vi "MGI Determine Time Format String.vi"(8 "error in (no error)":errorcluster, 9 "Day Before Month? (F)":bool, 10 "Leading Zeros? (F)":bool, 11 "DateTime String":string) -> (0 "error out":errorcluster, 3 "DateTime Format":string)   [LabVIEW 2016]
doc: "Determines a Time Format String for a given string in a common date format. For example Thu, January 1, 2011 3:00 PM would be %a, %B, %#d, %Y %#I:%M %p. The <b>Day Before Month?</b> input specifies whether the day or month is first when in a 12/1/11 type format. The <b>Leading Zeros?</b> input determines if the day, month number, and hour will have a leading zero if they are only 1 digit.\n\nAuthored by Hope Harrison\nsupport@mooregoodideas.com\nwww.mooregoodideas.com\n\nCopyright (c) 2010, Moore Good Ideas, Inc.\n\nAll rights reserved.\n\nRedistribution and use in source and binary forms, with or without modification, are permitted provided that the following conditions are met:\n\n * Redistributions of source code must retain the above copyright notice, this list of conditions and the following disclaimer.\n * Redistributions in binary form must reproduce the above copyright notice, this list of conditions and the following disclaimer in the documentation and/or other materials provided with the distribution.\n * Neither the name of Moore Good Ideas, Inc. nor the names of its contributors may be used to endorse or promote products derived from this software without specific prior written permission.\n\nTHIS SOFTWARE IS PROVIDED BY THE COPYRIGHT HOLDERS AND CONTRIBUTORS \"AS IS\" AND ANY EXPRESS OR IMPLIED WARRANTIES, INCLUDING, BUT NOT LIMITED TO, THE IMPLIED WARRANTIES OF MERCHANTABILITY AND FITNESS FOR A PARTICULAR PURPOSE ARE DISCLAIMED. IN NO EVENT SHALL THE COPYRIGHT OWNER OR CONTRIBUTORS BE LIABLE FOR ANY DIRECT, INDIRECT, INCIDENTAL, SPECIAL, EXEMPLARY, OR CONSEQUENTIAL DAMAGES (INCLUDING, BUT NOT LIMITED TO, PROCUREMENT OF SUBSTITUTE GOODS OR SERVICES; LOSS OF USE, DATA, OR PROFITS; OR BUSINESS INTERRUPTION) HOWEVER CAUSED AND ON ANY THEORY OF LIABILITY, WHETHER IN CONTRACT, STRICT LIABILITY, OR TORT (INCLUDING NEGLIGENCE OR OTHERWISE) ARISING IN ANY WAY OUT OF THE USE OF THIS SOFTWARE, EVEN IF ADVISED OF THE POSSIBILITY OF SUCH DAMAGE."
uses:
  <userlib>/_MGI/String/MGI Determine Time Format String/MGI Local Time Strings.ctl
  <userlib>/_MGI/String/MGI Determine Time Format String/MGI Parts of Date Found.ctl
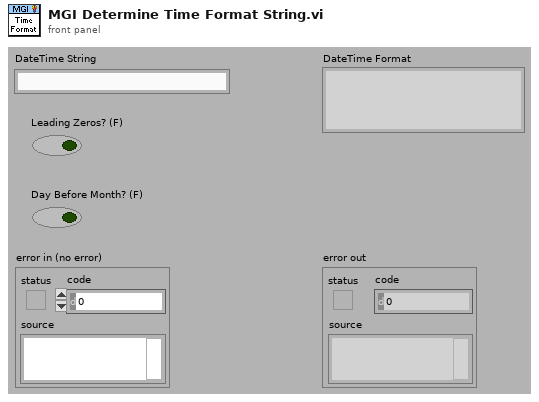
[diagram p1: front panel]
types:
  T1 = typedef "MGI Local Time Strings.ctl" = cluster{"Month[]":string[], "AMPM[]":string[], "Weekday[]":string[]}
  T2 = cluster{"fractional second":dbl, "second":i32, "minute":i32, "hour":i32, "day of month":i32, "month":i32, "year":i32, "day of week":i32, "day of year":i32, "DST":i32}
  T3 = typedef "MGI Parts of Date Found.ctl" = cluster{"Found Month?":bool, "Found Day?":bool, "Found Year?":bool}
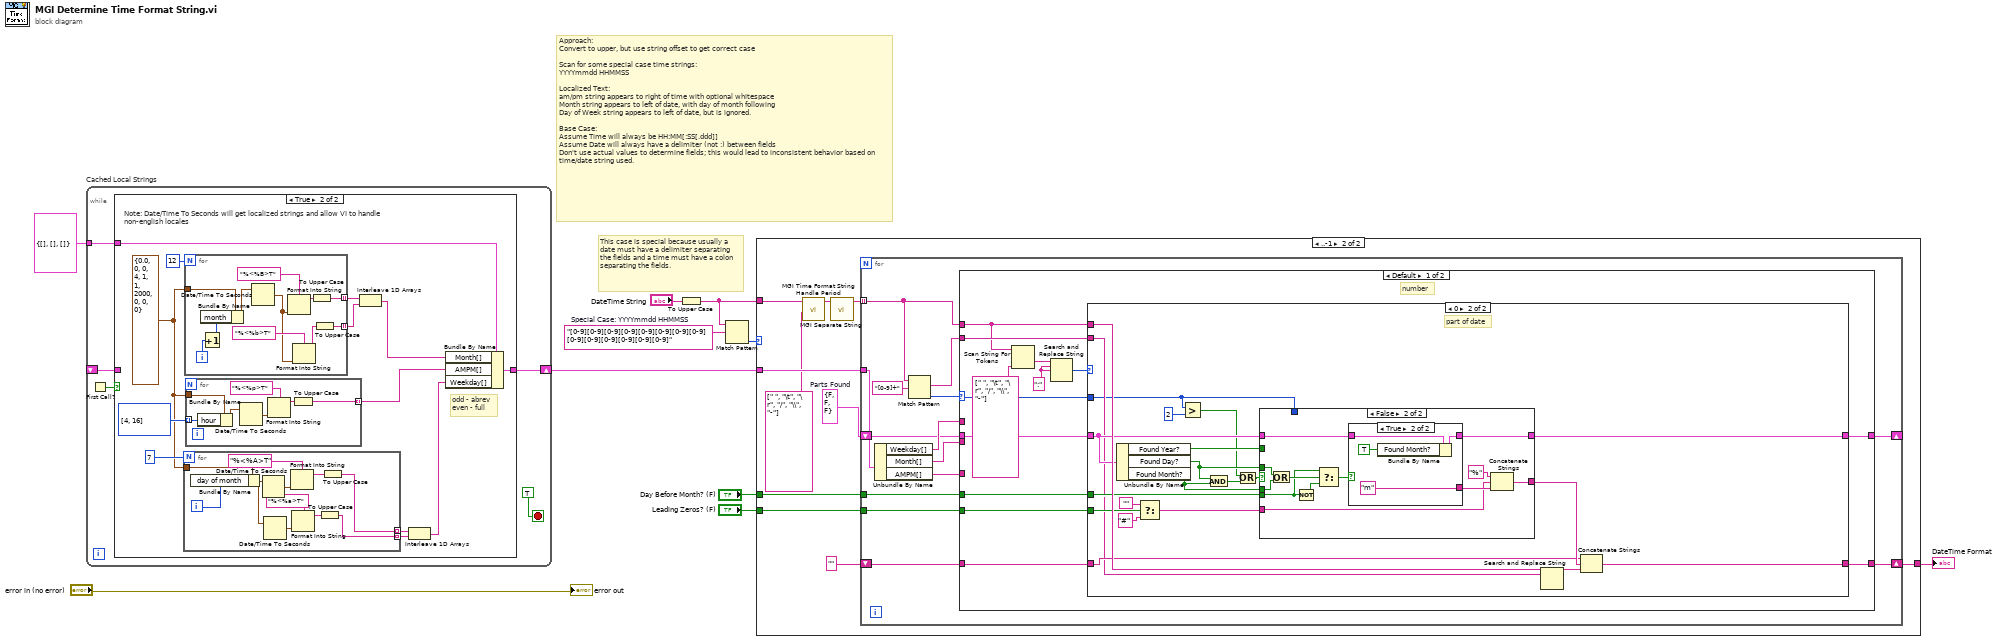
[diagram p0: block diagram]
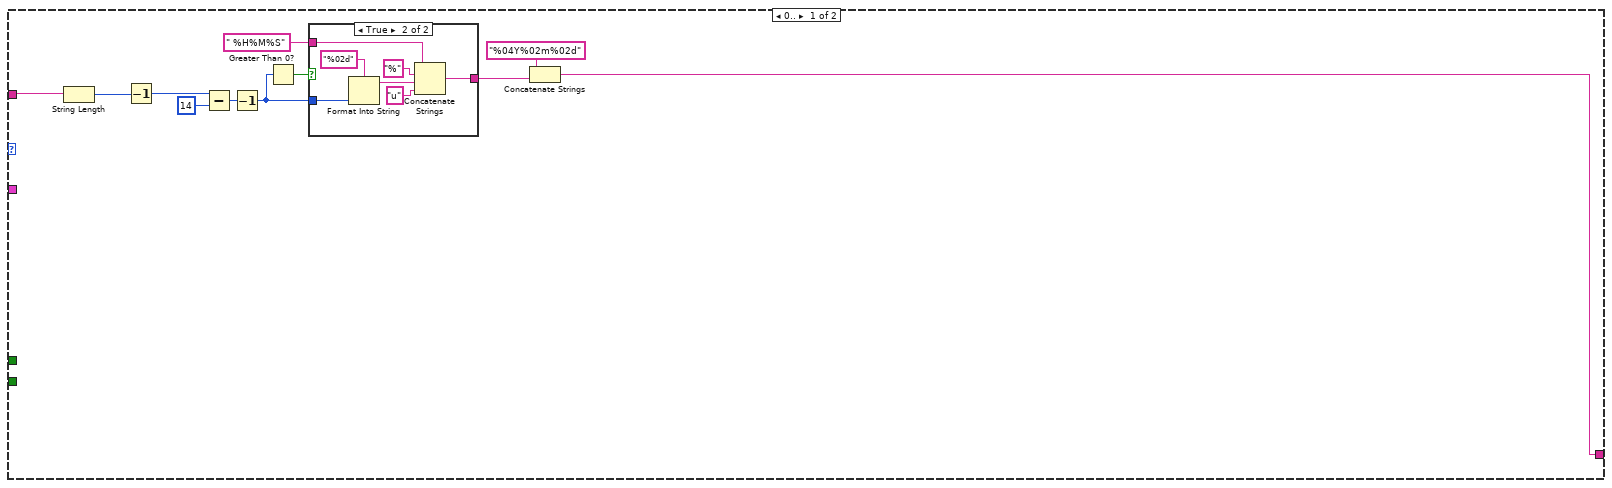
[diagram p2: hidden frame]
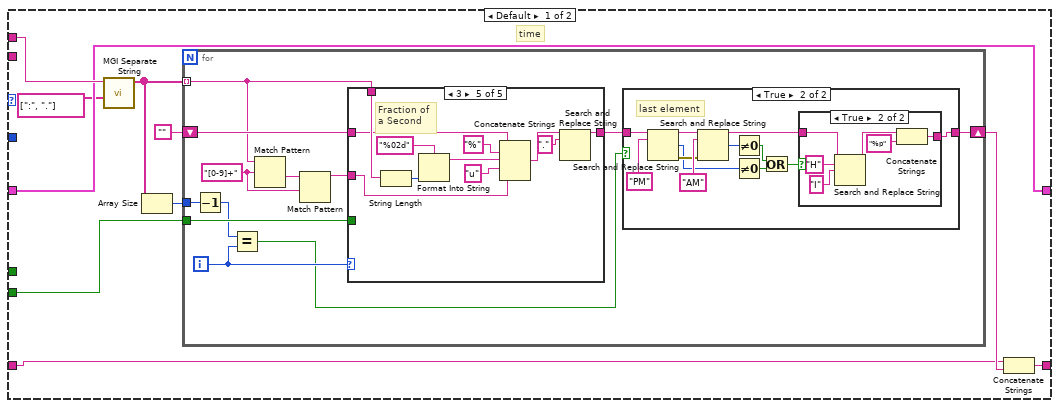
[diagram p4: hidden frame]
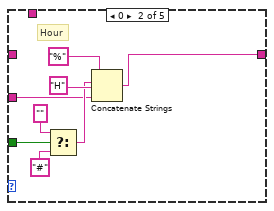
[diagram p8: hidden frame]
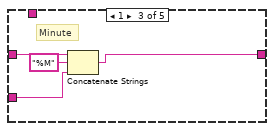
[diagram p9: hidden frame]
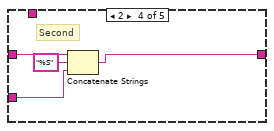
[diagram p10: hidden frame]
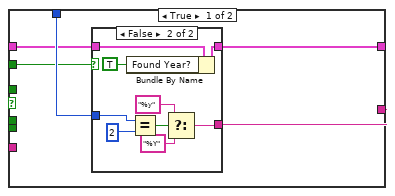
[diagram p11: hidden frame]
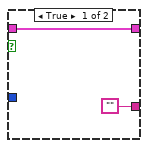
[diagram p12: hidden frame]
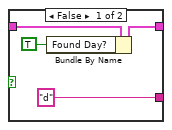
[diagram p13: hidden frame]
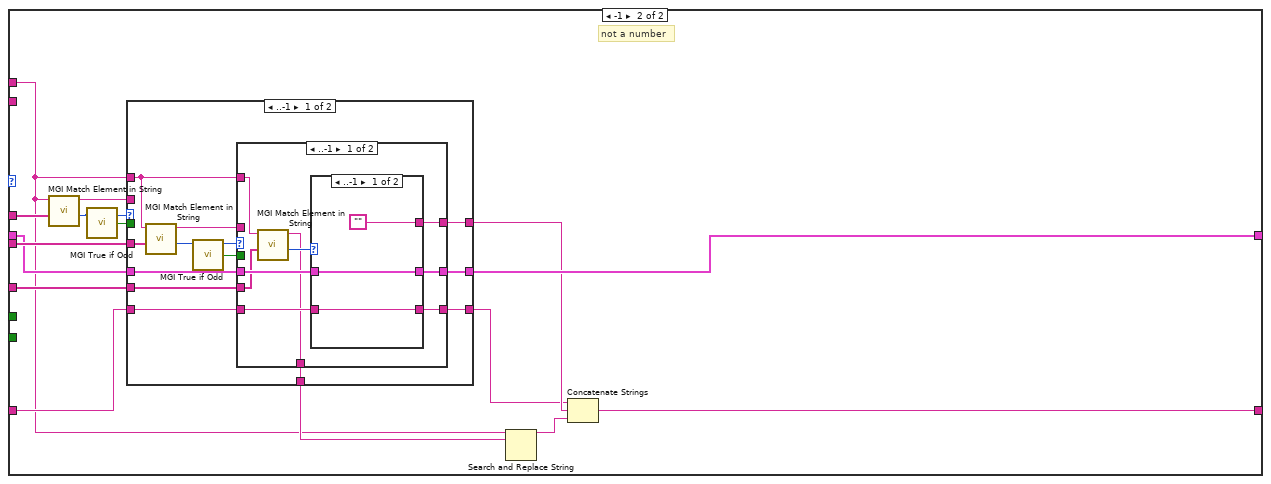
[diagram p14: hidden frame]
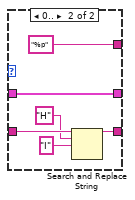
[diagram p15: hidden frame]
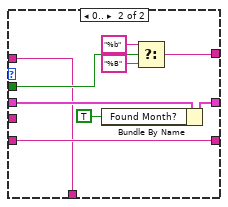
[diagram p16: hidden frame]
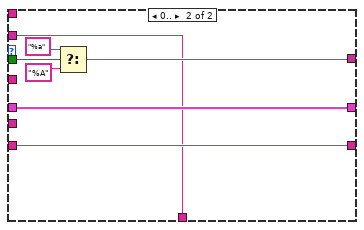
[diagram p17: hidden frame]
diagram:
  w8 = "[0-9][0-9][0-9][0-9][0-9][0-9][0-9][0-9] [0-9][0-9][0-9][0-9][0-9][0-9]"  # Special Case: YYYYmmdd HHMMSS
  # "This case is special because usually a date must have a delimiter separating the fields and a time must have a colon separating the fields."
  # "Approach:\nConvert to upper, but use string offset to get correct case\n\nScan for some special case time strings:\nYYYYmmdd HHMMSS\n\nLocalized Text:\nam/pm string appears to right of time with optional whitespace\nMonth string appears to left of date, with day of month following\nDay of Week string appears to left of date, but is ignored.\n\nBase Case:\nAssume Time will always be HH:MM[:SS[.ddd]]\nAssume Date will always have a delimiter (not :) between fields\nDon't use actual values to determine fields; this would lead to inconsistent behavior based on time/date string used."
  n1 = while "Cached Local Strings" {
    shift-right: [w13] -> w3
    shift-left: _ -> [w12]
    tunnel: T1 {"Month[]"=[], "AMPM[]"=[], "Weekday[]"=[]} ("cluster") -> [w11]
    stop <- TRUE stop-if-true
    n2 = First Call?() -> (First Call?: T/F=w14:bool)
    n3 = case shown="True" w14 {
      tunnel: [w16 w28] -> w13
      tunnel: w12 -> [w16 _]
      tunnel: w11 -> [_ w24]
      frame False {
      }
      frame True {
        w25 = T2 {"fractional second"=0.0, "second"=0, "minute"=0, "hour"=4, "day of month"=1, "month"=1, "year"=2000, "day of week"=0, "day of year"=0, "DST"=0} ("date time rec")
        # "odd - abrev\neven - full"
        # "Note: Date/Time To Seconds will get localized strings and allow VI to handle non-english locales"
        n4 = for {
          N: 7 -> [_]
          tunnel: w25 -> [w38]
          tunnel: [w31] -> w23 mode=indexing
          tunnel: [w30] -> w22 mode=indexing
          i -> [w36]
          n5 = Bundle By Name(cluster=w38, "day of month"=w36) -> (w34:T2)
          n6 = Date/Time To Seconds(2:w34) -> (0:w39:timestamp)  [unwired: 1 in]
          n7 = Date/Time To Seconds(2:w34) -> (0:w35:timestamp)  [unwired: 1 in]
          n8 = Format Into String(format string="%<%A>T", w39) -> (resulting string=w37:string)  [unwired: 2 in, 1 out]
          n9 = Format Into String(format string="%<%a>T", w35) -> (resulting string=w32:string)  [unwired: 2 in, 1 out]
          n10 = To Upper Case(1:w32) -> (0:w30:string)
          n11 = To Upper Case(1:w37) -> (0:w31:string)
        }
        n12 = for {
          N: 12 -> [_]
          tunnel: w25 -> [w55]
          tunnel: [w49] -> w20 mode=indexing
          tunnel: [w48] -> w19 mode=indexing
          i -> [w54]
          n13 = Increment(x=w54) -> (x+1=w52:i32)
          n14 = Bundle By Name(cluster=w55, "month"=w52) -> (w53:T2)
          n15 = Date/Time To Seconds(2:w53) -> (0:w56:timestamp)  [unwired: 1 in]
          n16 = Format Into String(format string="%<%B>T", w56) -> (resulting string=w51:string)  [unwired: 2 in, 1 out]
          n17 = Format Into String(format string="%<%b>T", w56) -> (resulting string=w50:string)  [unwired: 2 in, 1 out]
          n18 = To Upper Case(1:w51) -> (0:w49:string)
          n19 = To Upper Case(1:w50) -> (0:w48:string)
        }
        n20 = for {
          tunnel: w25 -> [w44]
          tunnel: i32[] [4, 16] -> [w43] mode=indexing
          tunnel: [w41] -> w17 mode=indexing
          n21 = Bundle By Name(cluster=w44, "hour"=w43) -> (w46:T2)
          n22 = Date/Time To Seconds(2:w46) -> (0:w45:timestamp)  [unwired: 1 in]
          n23 = Format Into String(format string="%<%p>T", w45) -> (resulting string=w42:string)  [unwired: 2 in, 1 out]
          n24 = To Upper Case(1:w42) -> (0:w41:string)
        }
        n25 = Interleave 1D Arrays(w20, w19) -> (w18:string[])
        n26 = Interleave 1D Arrays(w23, w22) -> (w21:string[])
        n27 = Bundle By Name(cluster=w24, "Month[]"=w18, "AMPM[]"=w17, "Weekday[]"=w21) -> (w28:T1)
      }
    }
  }
  n28 = To Upper Case(1:"DateTime String") -> (0:w6:string)
  n29 = Match Pattern(string=w6, regular expression=w8) -> (offset past match=w7:i32)  [unwired: 1 in, 3 out]
  n30 = case shown="..-1" w7 {
    tunnel: w6 -> [w69 w86]
    tunnel: "Leading Zeros? (F)" -> [_ w82]
    tunnel: "Day Before Month? (F)" -> [_ w81]
    tunnel: w3 -> [_ w83]
    tunnel: [w60 w84] -> w2
    frame 0.. {
      # "Special Case"
      n31 = String Length(string=w69) -> (length=w68:i32)
      n32 = Decrement(x=w68) -> (x-1=w63:i32)
      n33 = Subtract(x=w63, y=14 ("Date.Len")) -> (x-y=w66:i32)
      n34 = Decrement(x=w66) -> (x-1=w64:i32)
      n35 = Greater Than 0?(x=w64) -> (x > 0?=w67:bool)
      n36 = case shown="True" w67 {
        tunnel: w64 -> [_ w73]
        tunnel: " %H%M%S" ("Time.Format") -> [w70 w72]
        tunnel: [w70 w71] -> w62
        frame False {
        }
        frame True {
          n37 = Format Into String(format string="%02d", w73) -> (resulting string=w74:string)  [unwired: 2 in, 1 out]
          n38 = Concatenate Strings(w72, "%" ("string"), w74, "u" ("string")) -> (w71:string)
        }
      }
      n39 = Concatenate Strings("%04Y%02m%02d" ("Date.Format"), w62) -> (w60:string)
    }
    frame ..-1 {
      w85 = T3 {"Found Month?"=FALSE, "Found Day?"=FALSE, "Found Year?"=FALSE}  # Parts Found
      n40 = call <userlib>:"MGI Separate String.vi"("Separators"=string[] [" ", "\t", "\r", "/", "\\", "-"] ("delimiters (\\s,\\t,\\r,\\n)"), "String"=w86) -> ("Separated String"=w78:string[])  [unwired: 9 in]
      n41 = call <userlib>:"MGI Time Format String Handle Period.vi"("String[]"=w78) -> ("Separated String[]"=w80:string[])  [unwired: 10 in]
      n42 = for {
        tunnel: w83 -> [w101]
        shift-right: [w91] -> w84
        shift-left: "" -> [w92]
        tunnel: w80 -> [w100] mode=indexing
        shift-right: [w94] -> _
        shift-left: w85 -> [w95]
        tunnel: w82 -> [w89]
        tunnel: w81 -> [w88]
        n43 = Unbundle By Name(w101) -> ("Weekday[]"=w97:string[], "Month[]"=w96:string[], "AMPM[]"=w90:string[])
        n44 = Match Pattern(string=w100, regular expression="[0-9]+") -> (match substring=w93:string, offset past match=w98:i32)  [unwired: 1 in, 2 out]
        n45 = case shown="Default" w98 {
          selector: w98 -> [w113 _]
          tunnel: w100 -> [w106 w244]
          tunnel: w97 -> [_ w245]
          tunnel: w96 -> [_ w256]
          tunnel: w95 -> [w112 w255]
          tunnel: [w114 w253] -> w94
          tunnel: w93 -> [w107 _]
          tunnel: w92 -> [w105 w248]
          tunnel: [w104 w250] -> w91
          tunnel: w90 -> [_ w249]
          tunnel: w89 -> [w103 _]
          tunnel: w88 -> [w102 _]
          frame Default {
            w109 = ":"
            # "number"
            n46 = Scan String For Tokens(6:string[] [" ", "\t", "\r", "/", "\\", "-"] ("delimiters (\\s,\\t,\\r,\\n)"), 9:w106) -> (1:w110:string)  [unwired: 4 in, 3 out]
            n47 = Search and Replace String(input string=w110, search string=w109, replace string=w109) -> (number of replacements=w108:i32)  [unwired: 5 in, 3 out]
            n48 = case shown="0" w108 {
              tunnel: [w118 w200] -> w114
              tunnel: w113 -> [_ w187]
              tunnel: w112 -> [w118 w201]
              tunnel: w107 -> [_ w188]
              tunnel: w106 -> [w122 w204]
              tunnel: w105 -> [w120 w197]
              tunnel: [w121 w202] -> w104
              tunnel: w103 -> [w119 w192]
              tunnel: w102 -> [_ w190]
              frame Default {
                # "time"
                n49 = call <userlib>:"MGI Separate String.vi"("Separators"=string[] [":", "."], "String"=w122) -> ("Separated String"=w117:string[])  [unwired: 9 in]
                n50 = Array Size(array=w117) -> (size(s)=w116:i32)
                n51 = for {
                  tunnel: w117 -> [w125] mode=indexing
                  tunnel: w119 -> [w136]
                  shift-right: [w126] -> w123
                  shift-left: "" -> [w135]
                  tunnel: w116 -> [w131]
                  i -> [w129]
                  w134 = "[0-9]+" ("regular expression")
                  n52 = Decrement(x=w131) -> (x-1=w130:i32)
                  n53 = Equal?(x=w130, y=w129) -> (x = y?=w128:bool)
                  n54 = Match Pattern(string=w125, regular expression=w134) -> (after substring=w133:string)  [unwired: 1 in, 3 out]
                  n55 = Match Pattern(string=w133, regular expression=w134) -> (before substring=w132:string)  [unwired: 1 in, 3 out]
                  n56 = case shown="3" w129 {
                    tunnel: w136 -> [_ w165 _ _ _]
                    tunnel: [w157 w161 w167 w171 w175] -> w127
                    tunnel: w135 -> [w157 _ w169 w173 w178]
                    tunnel: w125 -> [_ _ _ _ w181]
                    tunnel: w132 -> [_ w158 w166 w170 w177]
                    frame Default {
                      (unwired) 0
                    }
                    frame 0 {
                      # "Hour"
                      n57 = Select(t="", s=w165, f="#") -> (s? t:f=w159:string)
                      n58 = Concatenate Strings("%" ("string"), w159, "H", w158) -> (w161:string)
                    }
                    frame 1 {
                      # "Minute"
                      n59 = Concatenate Strings(w169, "%M" ("string"), w166) -> (w167:string)
                    }
                    frame 2 {
                      # "Second"
                      n60 = Concatenate Strings(w173, "%S" ("string"), w170) -> (w171:string)
                    }
                    frame 3 {
                      # "Fraction of\na Second"
                      n61 = String Length(string=w181) -> (length=w180:i32)
                      n62 = Format Into String(format string="%02d", w180) -> (resulting string=w183:string)  [unwired: 2 in, 1 out]
                      n63 = Concatenate Strings(w178, "%" ("string"), w183, "u" ("string"), w177) -> (w176:string)
                      n64 = Search and Replace String(input string=w176, search string=".") -> (result string=w175:string)  [unwired: 6 in, 3 out]
                    }
                  }
                  n65 = case shown="True" w128 {
                    tunnel: [w137 w148] -> w126
                    tunnel: w127 -> [w137 w147]
                    frame False {
                    }
                    frame True {
                      # "last element"
                      n66 = Search and Replace String(input string=w147, search string="PM") -> (result string=w144:string, number of replacements=w142:i32, error out=w145:errorcluster)  [unwired: 6 in, 1 out]
                      n67 = Search and Replace String(input string=w144, search string="AM", error in=w145) -> (result string=w143:string, number of replacements=w141:i32)  [unwired: 5 in, 2 out]
                      n68 = Not Equal To 0?(x=w141) -> (x != 0?=w139:bool)
                      n69 = Not Equal To 0?(x=w142) -> (x != 0?=w140:bool)
                      n70 = Or(x=w139, y=w140) -> (x .or. y?=w138:bool)
                      n71 = case shown="True" w138 {
                        tunnel: [w150 w156] -> w148
                        tunnel: w143 -> [w150 w154]
                        frame False {
                        }
                        frame True {
                          n72 = Search and Replace String(input string=w154, search string="H", replace string="I" ("replace string (\"\")")) -> (result string=w153:string)  [unwired: 5 in, 3 out]
                          n73 = Concatenate Strings(w153, "%p" ("search string")) -> (w156:string)
                        }
                      }
                    }
                  }
                }
                n74 = Concatenate Strings(w120, w123) -> (w121:string)
              }
              frame 0 {
                # "part of date"
                n75 = Unbundle By Name(w201) -> ("Found Year?"=w193:bool, "Found Day?"=w195:bool, "Found Month?"=w191:bool)
                n76 = Select(t="", s=w192, f="#" ("regular expression")) -> (s? t:f=w196:string)
                n77 = Greater?(x=w187, y=2) -> (0:w185:bool)
                n78 = And(x=w195, y=w191) -> (x .and. y?=w194:bool)
                n79 = Or(x=w185, y=w194) -> (x .or. y?=w189:bool)
                n80 = case shown="False" w189 {
                  tunnel: [w207 w228] -> w203
                  tunnel: w201 -> [w208 w233]
                  tunnel: [w206 w229] -> w200
                  tunnel: w196 -> [_ w230]
                  tunnel: w195 -> [_ w227]
                  tunnel: w187 -> [w210 _]
                  tunnel: w193 -> [w209 _]
                  tunnel: w190 -> [_ w224]
                  tunnel: w191 -> [_ w222]
                  frame True {
                    n81 = case shown="False" w209 {
                      tunnel: w210 -> [_ w213]
                      tunnel: [w212 w215] -> w206
                      tunnel: w208 -> [w212 w216]
                      tunnel: ["" w214] -> w207
                      frame True {
                      }
                      frame False {
                        n82 = Bundle By Name(cluster=w216, "Found Year?"=TRUE ("ignore case? (F)")) -> (w215:T3)
                        n83 = Equal?(x=w213, y=2) -> (x = y?=w221:bool)
                        n84 = Select(t="%y" ("regular expression"), s=w221, f="%Y" ("regular expression")) -> (s? t:f=w214:string)
                      }
                    }
                  }
                  frame False {
                    n85 = Or(x=w227, y=w222) -> (x .or. y?=w226:bool)
                    n86 = Not(x=w224) -> (.not. x?=w225:bool)
                    n87 = Select(t=w224, s=w226, f=w225) -> (s? t:f=w223:bool)
                    n88 = case shown="True" w223 {
                      tunnel: w233 -> [w236 w240]
                      tunnel: [w235 w239] -> w229
                      tunnel: ["d" ("regular expression") "m" ("regular expression")] -> w231
                      frame False {
                        n89 = Bundle By Name(cluster=w236, "Found Day?"=TRUE ("ignore case? (F)")) -> (w235:T3)
                      }
                      frame True {
                        n90 = Bundle By Name(cluster=w240, "Found Month?"=TRUE ("ignore case? (F)")) -> (w239:T3)
                      }
                    }
                    n91 = Concatenate Strings("%" ("regular expression"), w230, w231) -> (w228:string)
                  }
                }
                n92 = Search and Replace String(input string=w204, search string=w188) -> (result string=w205:string)  [unwired: 6 in, 3 out]
                n93 = Concatenate Strings(w197, w203, w205) -> (w202:string)
              }
            }
          }
          frame -1 {
            # "not a number"
            n94 = call <userlib>:"MGI Match Element in String.vi"("Match[]"=w245, "String"=w244) -> ("Index"=w242:i32, "Match"=w243:string)  [unwired: 7 in, 1 out]
            n95 = call <userlib>:"MGI True if Odd.vi"("Integer"=w242) -> ("Odd?"=w254:bool)
            n96 = case shown="..-1" w242 {
              tunnel: w254 -> [_ w302]
              tunnel: w244 -> [w259 _]
              tunnel: w256 -> [w260 _]
              tunnel: [w268 w299] -> w251
              tunnel: w243 -> [_ w296]
              tunnel: w255 -> [w267 w298]
              tunnel: [w265 w298] -> w253
              tunnel: w249 -> [w264 _]
              tunnel: w248 -> [w263 w297]
              tunnel: [w262 w297] -> w247
              tunnel: [w261 w296] -> w246
              frame ..-1 {
                n97 = call <userlib>:"MGI Match Element in String.vi"("Match[]"=w260, "String"=w259) -> ("Index"=w258:i32, "Match"=w257:string)  [unwired: 7 in, 1 out]
                n98 = call <userlib>:"MGI True if Odd.vi"("Integer"=w258) -> ("Odd?"=w266:bool)
                n99 = case shown="..-1" w258 {
                  tunnel: w266 -> [_ w295]
                  tunnel: [w275 w292] -> w268
                  tunnel: w267 -> [w277 w291]
                  tunnel: [w276 w289] -> w265
                  tunnel: w259 -> [w271 _]
                  tunnel: w264 -> [w272 _]
                  tunnel: w263 -> [w274 w288]
                  tunnel: [w273 w288] -> w262
                  tunnel: w257 -> [_ w287]
                  tunnel: [w269 w287] -> w261
                  frame ..-1 {
                    n100 = call <userlib>:"MGI Match Element in String.vi"("Match[]"=w272, "String"=w271) -> ("Index"=w270:i32, "Match"=w269:string)  [unwired: 7 in, 1 out]
                    n101 = case shown="..-1" w270 {
                      tunnel: [w279 w286] -> w276
                      tunnel: w277 -> [w279 w286]
                      tunnel: ["" "%p"] -> w275
                      tunnel: [w278 w283] -> w273
                      tunnel: w274 -> [w278 w284]
                      frame ..-1 {
                      }
                      frame 0.. {
                        n102 = Search and Replace String(input string=w284, search string="H", replace string="I" ("replace string (\"\")")) -> (result string=w283:string)  [unwired: 5 in, 3 out]
                      }
                    }
                  }
                  frame 0.. {
                    n103 = Bundle By Name(cluster=w291, "Found Month?"=TRUE ("ignore case? (F)")) -> (w289:T3)
                    n104 = Select(t="%b" ("regular expression"), s=w295, f="%B" ("regular expression")) -> (s? t:f=w292:string)
                  }
                }
              }
              frame 0.. {
                n105 = Select(t="%a" ("regular expression"), s=w302, f="%A") -> (s? t:f=w299:string)
              }
            }
            n106 = Search and Replace String(input string=w244, search string=w246) -> (result string=w252:string)  [unwired: 6 in, 3 out]
            n107 = Concatenate Strings(w247, w251, w252) -> (w250:string)
          }
        }
      }
    }
  }
  "DateTime Format" <- w2
  "error out" <- "error in (no error)"
